vi "createConfigFilePath.vi"(8 "error in (no error)":errorcluster) -> (0 "error out":errorcluster, 3 "ConfigFilePath":path)   [LabVIEW 2018]
doc: "Create the path of default.ini file.\n\nNOTE: this is only for internal use. User does not call this function directly."
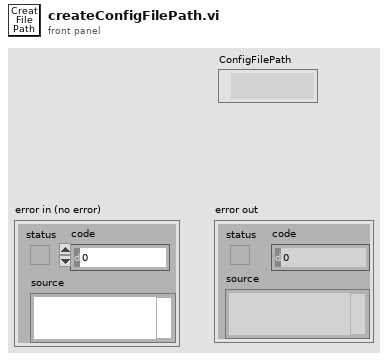
[diagram p1: front panel]
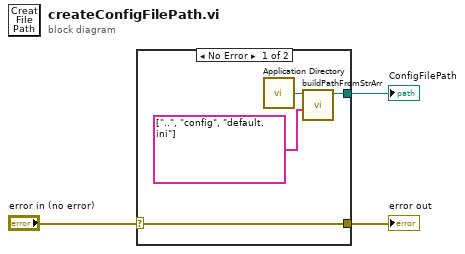
[diagram p0: block diagram]
diagram:
  n1 = case shown="No Error" "error in (no error)" {
    selector: "error in (no error)" -> [w7 w8]
    tunnel: [w7 w8] -> w2
    tunnel: [w4 _] -> w1
    frame No Error {
      n2 = call <vilib>:"Application Directory.vi"() -> ("Application Directory"=w6:path)
      n3 = call "buildPathFromStrArr.vi"("String Array"=string[] ["..", "config", "default.ini"], "Root Path"=w6) -> ("Absolute Path"=w4:path)  [unwired: 9 in]
    }
    frame Error {
    }
  }
  "error out" <- w2
  "ConfigFilePath" <- w1
